vi "LogCfg.vi"(6 "SensType":i32(ring) items=["No Sensor", "Photo", "Thermo", "Pyro"], 7 "FastIn":bool caption="Fast Logging to File\n(w/o display update)", 8 "FileIn":bool caption="Select Log File", 9 "AveragingIn":i32=100 caption="Averaging" min=1 max=999999 step=1, 10 "IntervalIn":dbl=1.0 caption="Interval Time [s]" min=0.1 max=9999.9 step=0.1 format="%.1f", 11 "SamplesIn":i32=1000 caption="No of Samples" min=2) -> (0 "FileOut":bool, 1 "AveragingOut":i32, 2 "IntervalOut":dbl, 3 "SamplesOut":i32, 4 "FastOut":bool, 5 "FileRefnum":refnum<file>)   [LabVIEW 2015]
panel:
  out "days":i16
  out "hh":i16
  out "mm":i16
  out "ss":i16
  out "Est Tm":dbl
  out "error out":errorcluster
  in  "stop":bool
  # "Configure Data Logging"
  # "- No of Samples\n- Averaging Rate\n- Interval\n- File"
  # "Duration"
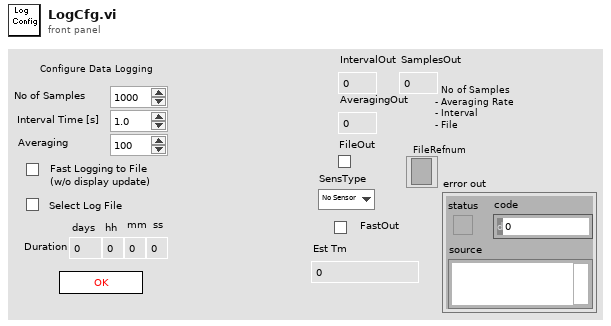
[diagram p1: front panel]
types:
  T1 = enum16{"open", "replace", "create", "open or create", "replace or create", "replace or create with confirmation"}
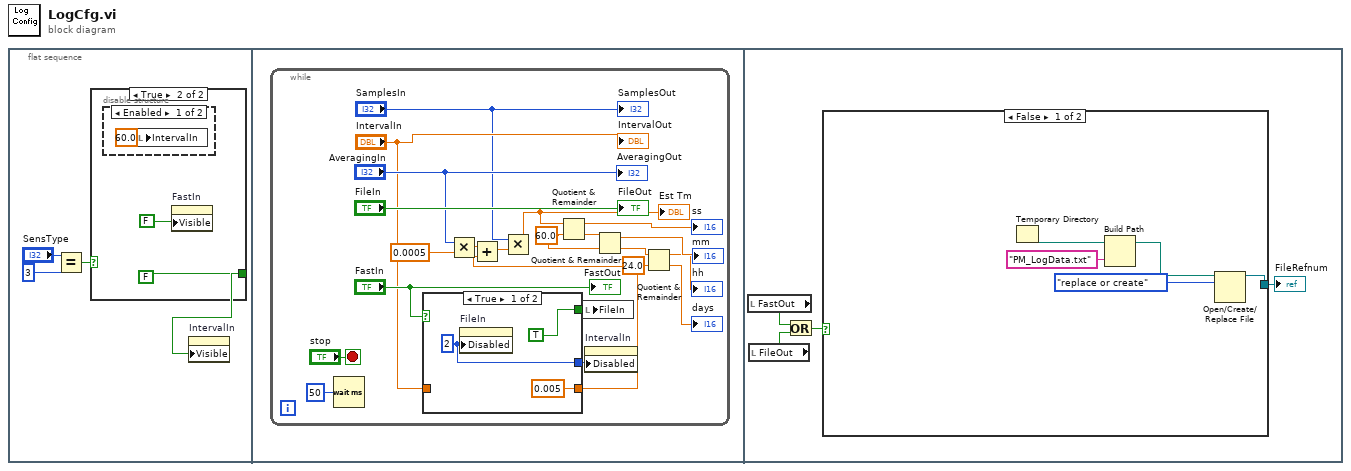
[diagram p0: block diagram]
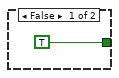
[diagram p2: hidden frame]
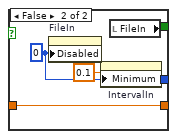
[diagram p4: hidden frame]
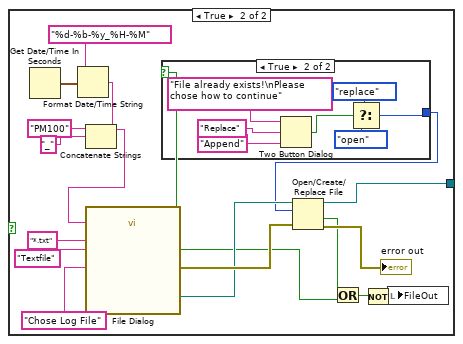
[diagram p5: hidden frame]
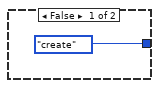
[diagram p6: hidden frame]
diagram:
  n1 = flat-sequence {
    frame #0 {
      n2 = Equal?(x="SensType", y=3) -> (x = y?=w2:bool)
      n3 = case shown="True" w2 {
        tunnel: [TRUE ("Visible") FALSE ("Visible")] -> w1
        frame False {
        }
        frame True {
          n4 = disable-structure shown="Enabled" {
            frame Enabled {
              n5 = local write "IntervalIn"(60.0 ("IntervalIn")) -> ()
            }
            frame Disabled {
            }
          }
          n6 = property on="FastIn" class="Bool (strict)"("Visible"=FALSE) -> ()  [unwired: 2 in, 2 out]
        }
      }
      n7 = property on="IntervalIn" class="DigNum (strict)"("Visible"=w1) -> ()  [unwired: 2 in, 2 out]
    }
    frame #1 {
      n8 = while {
        stop <- "stop" stop-if-true
        w14 = 60.0 ("y")
        n9 = Wait (ms)(milliseconds to wait=u32 50) -> ()  [unwired: 1 out]
        n10 = case shown="True" "FastIn" {
          tunnel: [TRUE w37] -> w26
          tunnel: [w32 w36] -> w25
          tunnel: [0.005 ("IntervalIn") w34] -> w20
          tunnel: "IntervalIn" -> [_ w34]
          frame True {
            w32 = u8 2 ("Disabled")
            n11 = property on="FileIn" class="Bool (strict)"("Disabled"=w32) -> ()  [unwired: 2 in, 2 out]
          }
          frame False {
            w36 = u8 0 ("Disabled")
            n12 = property on="FileIn" class="Bool (strict)"("Disabled"=w36) -> ()  [unwired: 2 in, 2 out]
            n13 = property on="IntervalIn" class="DigNum (strict)"("Minimum"=0.1 ("Data Entry Limits:Minimum")) -> ()  [unwired: 2 in, 2 out]
            n14 = local read "FileIn"() -> (w37:bool)
          }
        }
        n15 = Multiply(x="AveragingIn", y=0.0005 ("Data Entry Limits:Minimum")) -> (x*y=w21:dbl)
        n16 = Add(x=w21, y=w20) -> (x+y=w19:dbl)
        n17 = Multiply(x="SamplesIn", y=w19) -> (x*y=w17:dbl)
        "Est Tm" <- w17
        n18 = Quotient & Remainder(x=w17, y=w14) -> (x-y*floor(x/y)=→"ss":dbl, floor(x/y)=w15:dbl)
        n19 = local write "FileIn"(w26) -> ()
        n20 = property on="IntervalIn" class="DigNum (strict)"("Disabled"=w25) -> ()  [unwired: 2 in, 2 out]
        n21 = Quotient & Remainder(x=w15, y=w14) -> (x-y*floor(x/y)=→"mm":dbl, floor(x/y)=w12:dbl)
        n22 = Quotient & Remainder(x=w12, y=24.0) -> (x-y*floor(x/y)=→"hh":dbl, floor(x/y)=→"days":dbl)
        "IntervalOut" <- "IntervalIn"
        "SamplesOut" <- "SamplesIn"
        "AveragingOut" <- "AveragingIn"
        "FileOut" <- "FileIn"
        "FastOut" <- "FastIn"
      }
    }
    frame #2 {
      n23 = local read "FastOut"() -> (w40:bool)
      n24 = local read "FileOut"() -> (w39:bool)
      n25 = Or(x=w40, y=w39) -> (x .or. y?=w41:bool)
      n26 = case shown="False" w41 {
        tunnel: [w46 w47] -> w38
        frame False {
          n27 = Temporary Directory() -> (w42:path)
          n28 = Build Path(base path=w42, name or relative path="PM_LogData.txt") -> (appended path=w43:path)
          n29 = Open/Create/Replace File(file path (use dialog)=w43, operation (0:open)=T1."replace or create") -> (refnum out=w46:refnum<file>)  [unwired: 4 in, 2 out]
        }
        frame True {
          n30 = Get Date/Time In Seconds() -> (seconds since 1Jan1904=w53:timestamp)
          n31 = Format Date/Time String(time format string (%c)="%d-%b-%y_%H-%M", seconds (now)=w53) -> (date/time string=w50:string)  [unwired: 1 in]
          n32 = Concatenate Strings("PM100" ("default name"), "_" ("string"), w50) -> (w54:string)
          n33 = call "File Dialog"("prompt"="Chose Log File", "default name"=w54, "pattern (all files)"="*.txt", "pattern label"="Textfile" ("button label")) -> ("selected path"=w62:path, "exists"=w49:bool, "cancelled"=w58:bool, "error out"=w63:errorcluster)  [unwired: 8 in]
          n34 = case shown="True" w49 {
            tunnel: [T1."create" ("operation (0:open)") w67] -> w48
            frame False {
            }
            frame True {
              n35 = Two Button Dialog(message="File already exists!\nPlease chose how to continue", 1:"Append" ("F button name (\"Cancel\")"), 2:"Replace" ("T button name (\"OK\")")) -> (T button?=w69:bool)
              n36 = Select(t=T1."replace" ("operation (0:open)"), s=w69, f=T1."open" ("operation (0:open)")) -> (s? t:f=w67:T1)
            }
          }
          n37 = Open/Create/Replace File(file path (use dialog)=w62, error in=w63, operation (0:open)=w48) -> (refnum out=w47:refnum<file>, cancelled=w56:bool, error out=→"error out":errorcluster)  [unwired: 3 in]
          n38 = Or(x=w56, y=w58) -> (x .or. y?=w57:bool)
          n39 = Not(x=w57) -> (.not. x?=w65:bool)
          n40 = local write "FileOut"(w65) -> ()
        }
      }
      "FileRefnum" <- w38
    }
  }
